vi "Acquire Linearity Readings.vi"(5 "start label":string, 6 "Digital command info":T1, 7 "waveform name":string, 8 "error in":errorcluster, 9 "measure call context in":refnum<class "Measure Call Context.lvclass">, 10 "DMM session":refnum<k15>, 11 "Digital session":refnum<k15>) -> (0 "error out":errorcluster, 1 "measurement results":T2, 2 "DMM session out":refnum<k15>, 3 "Digital session out":refnum<k15>)   [LabVIEW 2021, in "Linearity_DAC.lvlib"]
uses:
  Linearity_DAC.lvlib
  <vilib>/MeasurementLink/MeasurementLink Measurement Server/Measure Call Context/Measure Call Context.lvclass
  Measurement Results.ctl
  <instrlib>/niDigital/niDigital.llb/niDigital Write Source Waveform (Broadcast U32).vi
  <instrlib>/niDigital/niDigital.llb/niDigital Burst Pattern (Pass Fail).vi
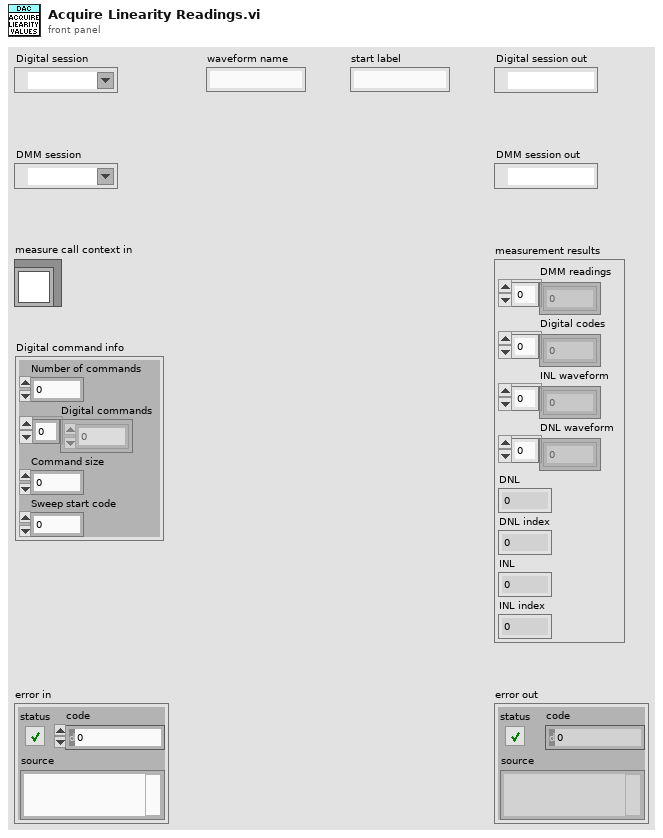
[diagram p1: front panel]
types:
  T1 = cluster{"Number of commands":u16, "Digital commands":i16[], "Command size":u16, "Sweep start code":u32}
  T2 = typedef "Linearity_DAC.lvlib/Measurement Results.ctl" = cluster{"DMM readings":dbl[], "Digital codes":u32[], "INL waveform":dbl[], "DNL waveform":dbl[], "DNL":dbl, "DNL index":u32, "INL":dbl, "INL index":u32}
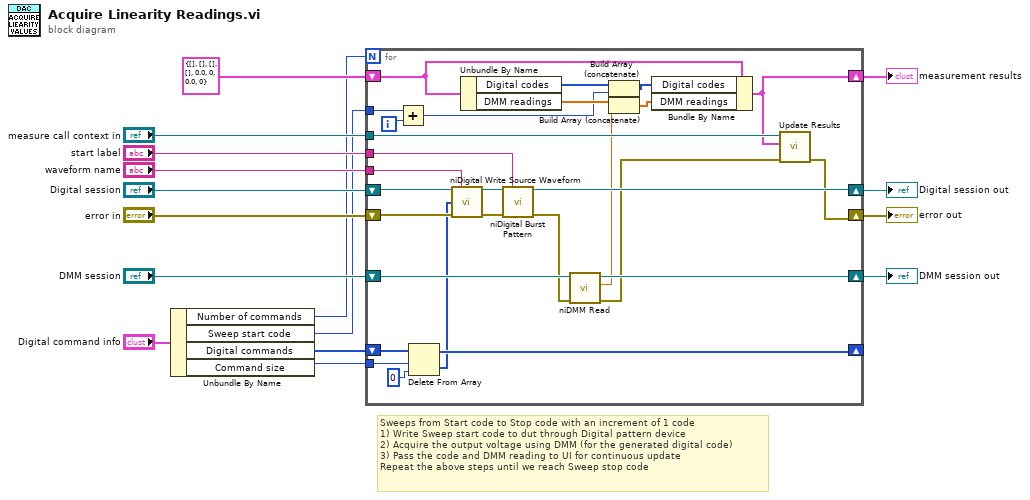
[diagram p0: block diagram]
diagram:
  # "Sweeps from Start code to Stop code with an increment of 1 code\n1) Write Sweep start code to dut through Digital pattern device\n2) Acquire the output voltage using DMM (for the generated digital code)\n3) Pass the code and DMM reading to UI for continuous update\nRepeat the above steps until we reach Sweep stop code"
  n1 = Unbundle By Name("Digital command info") -> ("Number of commands"=w1:u16, "Sweep start code"=w2:u32, "Digital commands"=w4:i16[], "Command size"=w3:u16)
  n2 = for {
    N: w1 -> [_]
    tunnel: w3 -> [w43]
    shift-right: [w40] -> _
    shift-left: w4 -> [w44]
    shift-right: [w37] -> w12
    shift-left: "Digital session" -> [w42]
    shift-right: [w17] -> w13
    shift-left: "error in" -> [w41]
    tunnel: "start label" -> [w36]
    shift-right: [w34] -> w14
    shift-left: "DMM session" -> [w35]
    tunnel: "waveform name" -> [w33]
    tunnel: "measure call context in" -> [w29]
    shift-right: [w24] -> w6
    shift-left: T2 {"DMM readings"=[], "Digital codes"=[], "INL waveform"=[], "DNL waveform"=[], "DNL"=0.0, "DNL index"=0, "INL"=0.0, "INL index"=0} ("measurement results") -> [w26]
    tunnel: w2 -> [w21]
    i -> [w20]
    n3 = Add(x=w21, y=w20) -> (x+y=w19:u32)
    n4 = Delete From Array(array=w44, length=w43, index=0) -> (deleted portion=w32:i16[], array with subset deleted=w40:i16[])
    n5 = call-poly <instrlib>:"niDigital Write Source Waveform.vi"("instrument handle"=w42, "waveform name"=w33, "waveform data"=w32, "error in"=w41) -> ("instrument handle out"=w39:refnum<k15>, "error out"=w38:errorcluster)  [unwired: 10 in]
    n6 = Unbundle By Name(w26) -> ("Digital codes"=w23:u32[], "DMM readings"=w27:dbl[])
    n7 = call-poly <instrlib>:"niDigital Burst Pattern.vi"("instrument handle"=w39, "start label"=w36, "error in"=w38) -> ("instrument handle out"=w37:refnum<k15>, "error out"=w30:errorcluster)  [unwired: 10 in, 1 out]
    n8 = call <instrlib>:"niDMM Read.vi"("error in (no error)"=w30, "instrument handle"=w35) -> ("error out"=w18:errorcluster, "Measurement"=w28:dbl, "instrument handle out"=w34:refnum<k15>)  [unwired: 7 in]
    n9 = Build Array (concatenate)(w23, w19) -> (w22:u32[])
    n10 = Build Array (concatenate)(w27, w28) -> (w25:dbl[])
    n11 = Bundle By Name(cluster=w26, "Digital codes"=w22, "DMM readings"=w25) -> (w24:T2)
    n12 = call <vilib>:"Update Results.vi"("error in"=w18, "measurement results"=w24, "measure call context in"=w29) -> ("error out"=w17:errorcluster)  [unwired: 7 in, 1 out]
  }
  "DMM session out" <- w14
  "error out" <- w13
  "Digital session out" <- w12
  "measurement results" <- w6
